vi "Word_Insert_Table.vi"(0 "Document":refnum<k7>, 1 "Tables":refnum<k7>, 2 "font":T1 {"font size" format="%0.2f"; "strike through" items=["Unchanged", "Yes", "No"]; "underline" items=["Unchanged", "Yes", "No"]; "italic" items=["Unchanged", "Yes", "No"]; "bold" items=["Unchanged", "Yes", "No"]}, 3 "show grid lines":bool=TRUE, 5 "Table data":string[][](array[string]), 7 "Start":i32, 9 "End":i32, 11 "error in (no error)":errorcluster, 12 "Insertion point":u16(ring)=1 items=["begining of document", "end of document", "bookmark", "Custom"], 13 "Bookmark name":string, 14 "column width (1)":dbl format="%0.2f") -> (8 "Start out":i32, 10 "End out":i32, 15 "error out":errorcluster)   [LabVIEW 2010, in "NI_ReportGenerationToolkit.lvlib"]
uses:
  <vilib>/addons/_office/NI_ReportGenerationToolkit.lvlib
  <vilib>/addons/_office/_exclsub.llb/font.ctl
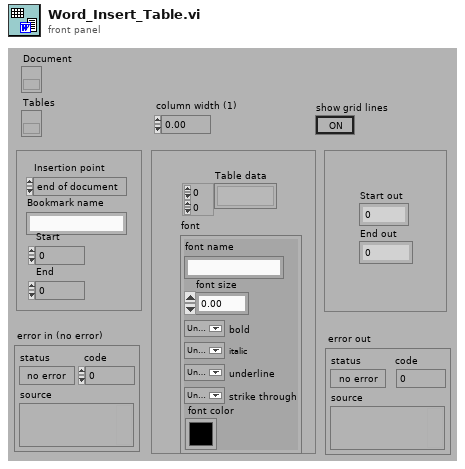
[diagram p1: front panel]
types:
  T1 = typedef "NI_ReportGenerationToolkit.lvlib/font.ctl" = cluster{"font name":string, "font size":dbl, "bold":u16, "italic":u16, "underline":u16, "strike through":u16, "font color":u32}
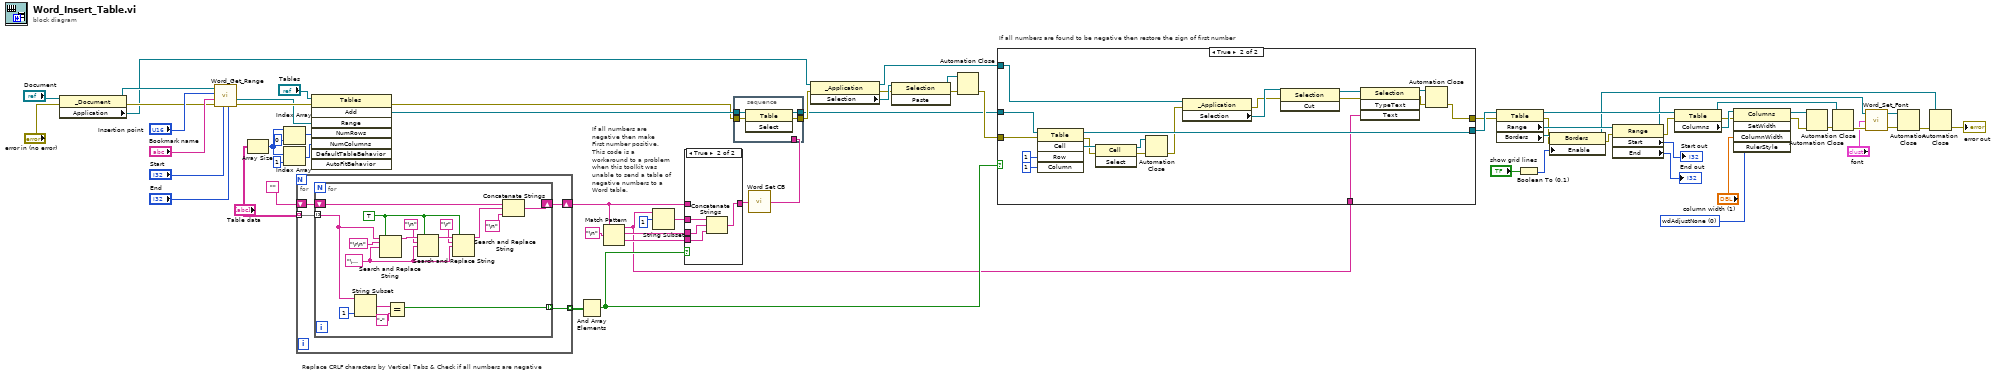
[diagram p0: block diagram]
diagram:
  w40 = 0 items=["wdAdjustNone", "wdAdjustProportional", "wdAdjustFirstColumn", "wdAdjustSameWidth"] ("RulerStyle")
  # "If all numbers are found to be negative then restore the sign of first number"
  # "If all numbers are negative then make\nFirst number positive. This code is a workaround to a problem when this toolkit was unable to send a table of negative numbers to a Word table."
  # "Replace CRLF characters by Vertical Tabs & Check if all numbers are negative"
  n1 = property class="_Document"(reference="Document", error in="error in (no error)") -> (reference out=w38:refnum<k7>, error out=w26:errorcluster, "Application"=w25:refnum<k7>)
  n2 = call <vilib>:"Word_Get_Range.vi"("end"="End", "start"="Start", "error in"=w26, "bookmark name"="Bookmark name", "insertion point"="Insertion point", "document in"=w38) -> ("error out (no error)"=w24:errorcluster, "range"=w23:refnum<k7>)  [unwired: 4 out]
  n3 = Array Size(array="Table data") -> (size(s)=w61:i32[])
  n4 = Index Array(array=w61, index=0 ("Indice")) -> (element=w58:i32)
  n5 = Index Array(array=w61, index=1 ("Indice")) -> (element=w57:i32)
  n6 = for {
    shift-right: [w71] -> w6
    shift-left: "" -> [w72]
    tunnel: "Table data" -> [w70] mode=indexing
    tunnel: [w69] -> w15 mode=indexing
    n7 = for {
      shift-right: [w87] -> w71
      shift-left: w72 -> [w88]
      tunnel: w70 -> [w77] mode=indexing
      tunnel: [w73] -> w69 mode=indexing
      w78 = TRUE ("replace all? (F)")
      w82 = "\u000b" ("replace string (\"\")")
      n8 = String Subset(string=w77, length (rest)=1 ("length (rest)")) -> (substring=w75:string)  [unwired: 1 out]
      n9 = Search and Replace String(replace all?=w78, input string=w77, search string="\r\n", replace string=w82) -> (result string=w84:string)  [unwired: 1 in, 6 out]
      n10 = Equal?(x=w75, y="-") -> (x = y?=w73:bool)
      n11 = Search and Replace String(replace all?=w78, input string=w84, search string="\n", replace string=w82) -> (result string=w83:string)  [unwired: 1 in, 6 out]
      n12 = Search and Replace String(replace all?=w78, input string=w83, search string="\r", replace string=w82) -> (result string=w81:string)  [unwired: 1 in, 6 out]
      n13 = Concatenate Strings(w88, w81, "\n") -> (w87:string)
    }
  }
  n14 = invoke class="Tables" method="Add"(reference="Tables", error in=w24, "Range"=w23, "NumRows"=w58, "NumColumns"=w57) -> (error out=w31:errorcluster, "Add"=w33:refnum<k7>)  [unwired: 3 in, 6 out]
  n15 = And Array Elements(Boolean array=w15) -> (logical AND=w8:bool)
  n16 = Match Pattern(string=w6, regular expression="\n") -> (before substring=w1:string, match substring=w3:string, after substring=w2:string)  [unwired: 2 out]
  n17 = String Subset(string=w1, offset (0)=1) -> (substring=w5:string)  [unwired: 1 out]
  n18 = case shown="True" w8 {
    tunnel: w6 -> [w89 _]
    tunnel: [w89 w93] -> w14
    tunnel: w5 -> [_ w92]
    tunnel: w3 -> [_ w91]
    tunnel: w2 -> [_ w90]
    frame False {
    }
    frame True {
      n19 = Concatenate Strings(w92, w91, w90) -> (w93:string)
    }
  }
  n20 = call <vilib>:"Word Set CB.vi"("String"=w14) -> ("String 2"=w16:string)
  n21 = stacked-sequence {
    tunnel: w33 -> [w97]
    tunnel: [w96] -> w12
    tunnel: w31 -> [w95]
    tunnel: [w94] -> w27
    tunnel: w16 -> [_]
    frame #0 {
      n22 = invoke class="Table" method="Select"(reference=w97, error in=w95) -> (reference out=w96:refnum<k7>, error out=w94:errorcluster)  [unwired: 1 in, 1 out]
    }
  }
  n23 = property class="_Application"(reference=w25, error in=w27) -> (reference out=w11:refnum<k7>, error out=w28:errorcluster, "Selection"=w32:refnum<k7>)
  n24 = invoke class="Selection" method="Paste"(reference=w32, error in=w28) -> (reference out=w29:refnum<k7>, error out=w30:errorcluster)  [unwired: 1 in, 1 out]
  n25 = Automation Close(3:w30, 5:w29) -> (0:w13:errorcluster)
  n26 = case shown="True" w8 {
    tunnel: w13 -> [w98 w114]
    tunnel: w12 -> [w99 w113]
    tunnel: w11 -> [_ w110]
    tunnel: [w99 w109] -> w10
    tunnel: [w98 w108] -> w9
    tunnel: w1 -> [_ w107]
    frame False {
    }
    frame True {
      n27 = invoke class="Table" method="Cell"(reference=w113, error in=w114, "Row"=1, "Column"=1) -> (reference out=w109:refnum<k7>, error out=w117:errorcluster, "Cell"=w118:refnum<k7>)  [unwired: 1 in, 2 out]
      n28 = invoke class="Cell" method="Select"(reference=w118, error in=w117) -> (reference out=w100:refnum<k7>, error out=w102:errorcluster)  [unwired: 1 in, 1 out]
      n29 = Automation Close(3:w102, 5:w100) -> (0:w101:errorcluster)
      n30 = property class="_Application"(reference=w110, error in=w101) -> (error out=w105:errorcluster, "Selection"=w106:refnum<k7>)  [unwired: 1 out]
      n31 = invoke class="Selection" method="Cut"(reference=w106, error in=w105) -> (reference out=w104:refnum<k7>, error out=w103:errorcluster)  [unwired: 1 in, 1 out]
      n32 = invoke class="Selection" method="TypeText"(reference=w104, error in=w103, "Text"=w107) -> (reference out=w115:refnum<k7>, error out=w116:errorcluster)  [unwired: 1 in, 2 out]
      n33 = Automation Close(3:w116, 5:w115) -> (0:w108:errorcluster)
    }
  }
  n34 = property class="Table"(reference=w10, error in=w9) -> (reference out=w50:refnum<k7>, error out=w54:errorcluster, "Range"=w66:refnum<k7>, "Borders"=w55:refnum<k7>)
  n35 = Boolean To (0,1)(Boolean="show grid lines") -> (0, 1=w51:i16)
  n36 = property class="Borders"(reference=w55, error in=w54, "Enable"=w51) -> (reference out=w46:refnum<k7>, error out=w53:errorcluster)
  n37 = property class="Range"(reference=w66, error in=w53) -> (reference out=w19:refnum<k7>, error out=w49:errorcluster, "Start"=→"Start out":i32, "End"=→"End out":i32)
  n38 = property class="Table"(reference=w50, error in=w49) -> (reference out=w45:refnum<k7>, error out=w43:errorcluster, "Columns"=w44:refnum<k7>)
  n39 = invoke class="Columns" method="SetWidth"(reference=w44, error in=w43, "ColumnWidth"="column width (1)", "RulerStyle"=w40) -> (reference out=w47:refnum<k7>, error out=w42:errorcluster)  [unwired: 1 in, 3 out]
  n40 = Automation Close(3:w42, 5:w47) -> (0:w48:errorcluster)
  n41 = Automation Close(3:w48, 5:w45) -> (0:w22:errorcluster)
  n42 = call <vilib>:"Word_Set_Font.vi"("Range in"=w19, "font"="font", "Error in"=w22) -> ("Range out"=w18:refnum<k7>, "Error out"=w21:errorcluster)  [unwired: 5 out]
  n43 = Automation Close(3:w21, 5:w18) -> (0:w20:errorcluster)
  n44 = Automation Close(3:w20, 5:w46) -> (0:→"error out":errorcluster)
